vi "Time_to_ms.vi"(2 "seconds since 1Jan1904":timestamp) -> (0 "Numeric":dbl)   [LabVIEW 2015]
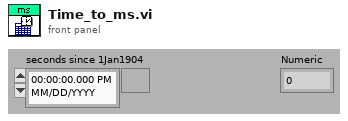
[diagram p1: front panel]
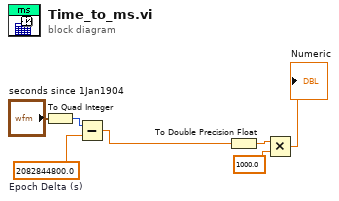
[diagram p0: block diagram]
diagram:
  w6 = 2082844800.0  # Epoch Delta (s)
  n1 = To Quad Integer(1:"seconds since 1Jan1904") -> (0:w2:i64)
  n2 = Subtract(x=w2, y=w6) -> (x-y=w1:dbl)
  n3 = To Double Precision Float(number=w1) -> (double precision float=w4:dbl)
  n4 = Multiply(x=w4, y=1000.0) -> (x*y=→"Numeric":dbl)
